vi "Builder.GetUserApp.vi"(8 "error in":errorcluster) -> (0 "error out":errorcluster, 3 "App Refnum":refnum<vi>)   [LabVIEW 2011]
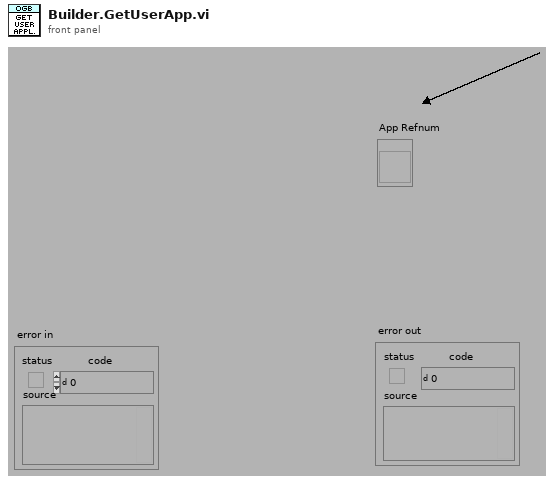
[diagram p1: front panel]
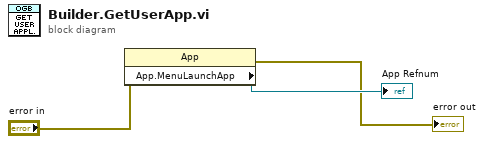
[diagram p0: block diagram]
diagram:
  n1 = property class="App"(error in="error in") -> (error out=→"error out":errorcluster, "App.MenuLaunchApp"=→"App Refnum":refnum<vi>)  [unwired: 1 in, 1 out]
